vi "TCE_Config_Load.vi"(8 "error in":errorcluster) -> (0 "error out":errorcluster, 3 "Config":T1={"Freezing"={"Cutoff"=2.0, "EndIndex"=2}})   [LabVIEW 2024]
uses:
  TCE_Config.ctl
  <vilib>/Utility/xml.llb/Read From XML File(string).vi
panel:
  in  "Default Values":T1={"Freezing"={"Cutoff"=2.0, "EndIndex"=2}}
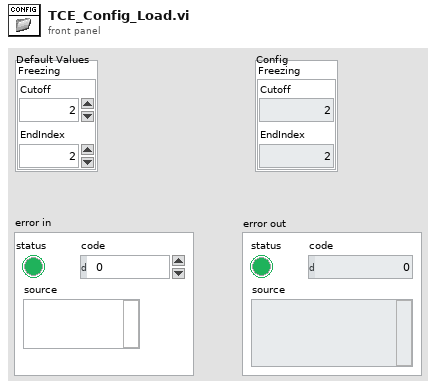
[diagram p1: front panel]
types:
  T1 = typedef "TCE_Config.ctl" = cluster{"Freezing":cluster{"Cutoff":dbl, "EndIndex":i32}}
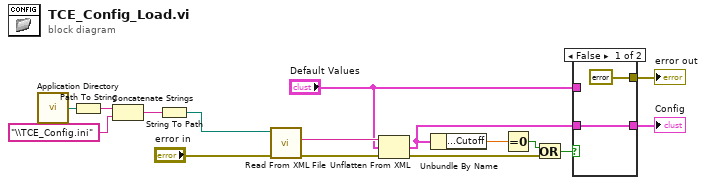
[diagram p0: block diagram]
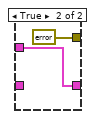
[diagram p2: hidden frame]
diagram:
  n1 = call <vilib>:"Application Directory.vi"() -> ("Application Directory"=w15:path)
  n2 = Path To String(path=w15) -> (string=w16:string)
  n3 = Concatenate Strings(w16, "\\TCE_Config.ini" ("string")) -> (w13:string)
  n4 = String To Path(string=w13) -> (path=w11:path)
  n5 = call-poly <vilib>:"Read From XML File.vi"("error in (no error)"="error in", "XML File Path"=w11) -> ("error out"=w9:errorcluster, "XML Elements"=w10:string)  [unwired: 7 in, 1 out]
  n6 = Unflatten From XML(xml string=w10, type="Default Values", error in (no error)=w9) -> (value=w7:T1, error out=w4:errorcluster)
  n7 = Unbundle By Name(w7) -> ("Freezing.Cutoff"=w8:dbl)
  n8 = Equal To 0?(x=w8) -> (x = 0?=w6:bool)
  n9 = Or(x=w6, y=w4) -> (x .or. y?=w5:bool)
  n10 = case shown="False" w5 {
    tunnel: [w18 w20] -> w1
    tunnel: "Default Values" -> [_ w20]
    tunnel: w7 -> [w18 _]
    tunnel: [errorcluster {"status"=FALSE, "code"=0, "source"=""} ("error in") errorcluster {"status"=FALSE, "code"=0, "source"=""} ("error in")] -> w3
    frame False {
    }
    frame True {
    }
  }
  "error out" <- w3
  "Config" <- w1
